vi "Configure Scale Band Math.vi"(0 "VISA resource name":refnum<visa-resource-name>, 1 "Lower Position (0)":i32, 2 "Upper Position (1)":i32=1, 5 "Channel (1)":string="001", 7 "Area (0 : Off)":i32(ring) items=["Off", "In", "Out"], 9 "Color":cluster{"R":i32, "G":i32, "B":i32} {"B" min=0 max=255 step=1; "G" min=0 max=255 step=1; "R" min=0 max=255 step=1}, 11 "error in (no error)":errorcluster) -> (4 "VISA resource name out":refnum<visa-resource-name>, 6 "Channel":string, 15 "error out":errorcluster)   [LabVIEW 2020, in "Yokogawa GX Series.lvlib"]
doc: "Sets the green band of math channel.\n\nCommand: SBandMath"
uses:
  <instrlib>/Yokogawa GX Series/Yokogawa GX Series.lvlib
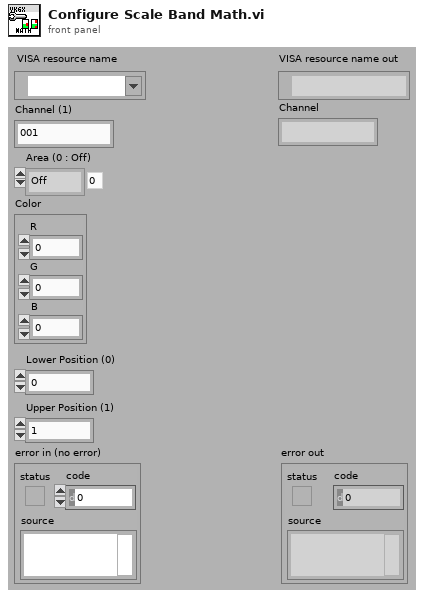
[diagram p1: front panel]
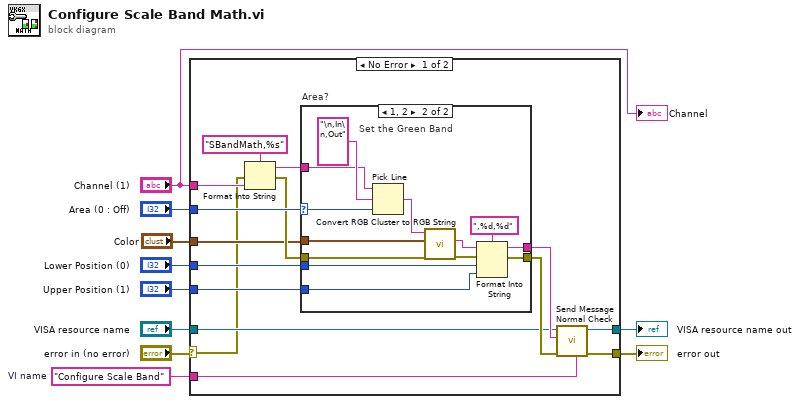
[diagram p0: block diagram]
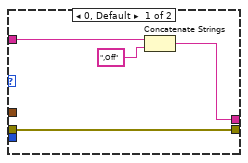
[diagram p2: hidden frame]
diagram:
  w10 = "Configure Scale Band"  # VI name
  n1 = case shown="No Error" "error in (no error)" {
    selector: "error in (no error)" -> [w11 w43]
    tunnel: w10 -> [w24 _]
    tunnel: "Area (0 : Off)" -> [w23 _]
    tunnel: "Lower Position (0)" -> [w20 _]
    tunnel: "Upper Position (1)" -> [w19 _]
    tunnel: "VISA resource name" -> [w16 w44]
    tunnel: [w15 w44] -> w5
    tunnel: [w14 w43] -> w4
    tunnel: "Color" -> [w13 _]
    tunnel: "Channel (1)" -> [w12 _]
    frame No Error {
      n2 = Format Into String(format string="SBandMath,%s", error in=w11, w12) -> (resulting string=w18:string, error out=w22:errorcluster)  [unwired: 1 in]
      n3 = case "Area?" shown="1, 2" w23 {
        selector: w23 -> [_ w36]
        tunnel: w22 -> [w29 w33]
        tunnel: [w29 w42] -> w21
        tunnel: w20 -> [_ w39]
        tunnel: w19 -> [_ w38]
        tunnel: [w26 w41] -> w17
        tunnel: w18 -> [w27 w35]
        tunnel: w13 -> [_ w34]
        frame 0, Default {
          n4 = Concatenate Strings(w27, ",Off") -> (w26:string)
        }
        frame 1, 2 {
          # "Set the Green Band"
          n5 = Pick Line(string ("")=w35, multi-line string="\n,In\n,Out" ("形式文字列"), line index=w36) -> (output string=w31:string)
          n6 = call <instrlib>:"Convert RGB Cluster to RGB String.vi"("error in (no error)"=w33, "RGB"=w34, "Initial String"=w31) -> ("error out"=w32:errorcluster, "RGB String"=w30:string)  [unwired: 7 in]
          n7 = Format Into String(format string=",%d,%d" ("形式文字列"), initial string=w30, error in=w32, w39, w38) -> (resulting string=w41:string, error out=w42:errorcluster)
        }
      }
      n8 = call <instrlib>:"Send Message Normal Check.vi"("Source (\"\")"=w24, "error in (no error)"=w21, "Send Message (\"\")"=w17, "VISA resource name"=w16) -> ("error out"=w14:errorcluster, "VISA resource name out"=w15:refnum<visa-resource-name>)  [unwired: 2 in, 4 out]
    }
    frame Error {
    }
  }
  "error out" <- w4
  "VISA resource name out" <- w5
  "Channel" <- "Channel (1)"
